vi "log.write_request.vi"(8 "error in":errorcluster, 9 "Arguments":map{string, string}(c390), 10 "Message":string, 11 "Time Stamp (now: system time)":timestamp format="%<%x %.3X>T") -> (0 "error out":errorcluster, 3 "request":string)   [LabVIEW 2020, in "Nominal Client.lvclass"]
uses:
  Nominal Client.lvclass
  4260bc31-df4d-47d5-a4e2-998131efb0a5.vi
  bb59544d-9623-4990-916d-6c8c801fc026.vi
  8accc981-0023-4d42-bd6a-63233f6e5657.vi
  <vilib>/LabVIEW Open Source Project/Epoch Date & Time/epoch.UNIX/Epoch.UNIX.lvclass
  C:/Program Files/National Instruments/LabVIEW 2020/vi.lib/LabVIEW Open Source Project/Epoch Date & Time/epoch/Epoch.lvclass
  <vilib>/LabVIEW Open Source Project/Epoch Date & Time/Get Epoch Time.vi
  <vilib>/JDP Science/JSONtext/Variant to JSON Text.vi
  <vilib>/JDP Science/JSONtext/support/Format JSON Object.vi
  <vilib>/JDP Science/JSONtext/LVClass Serializer/JSONtext LVClass Serializer.lvclass
  nominal types/properties/properties.lvclass
  Nominal Client.lvclass/Nominal Client.ctl
  <vilib>/JDP Science/JSONtext/JSONtext.lvlib
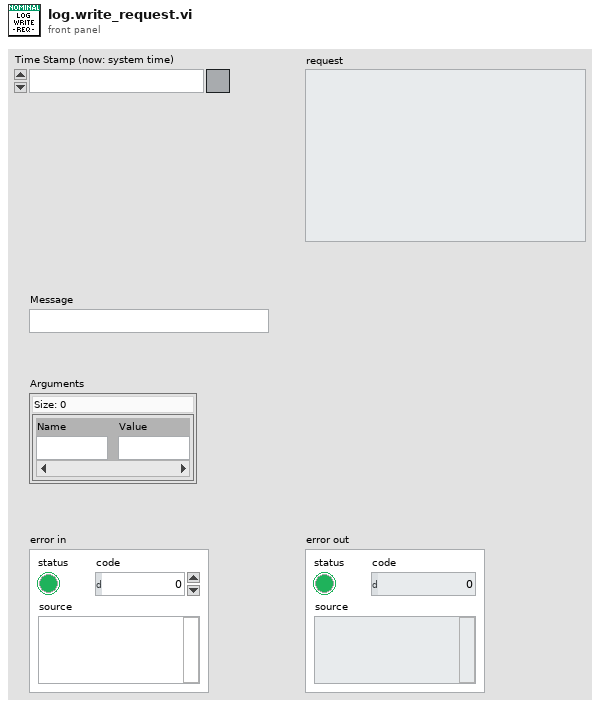
[diagram p1: front panel]
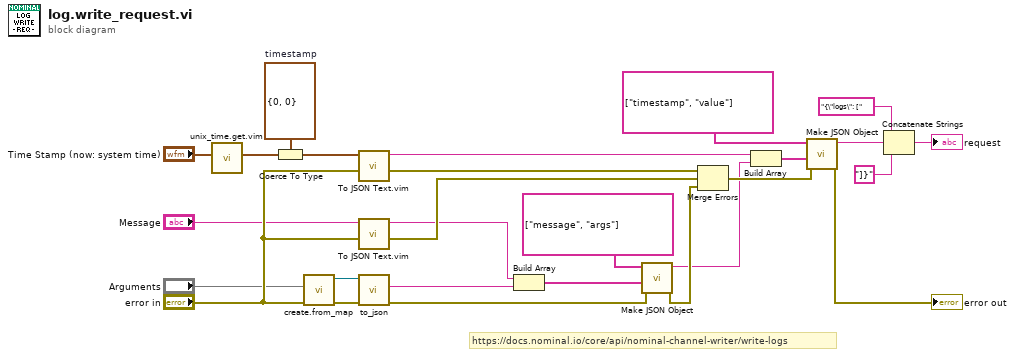
[diagram p0: block diagram]
diagram:
  w26 = cluster{"seconds":i32, "nanos":i32} {"seconds"=0, "nanos"=0}  # timestamp
  # "https://docs.nominal.io/core/api/nominal-channel-writer/write-logs"
  n1 = call "unix_time.get.vim"("Time Stamp (empty: now) [single or array]"="Time Stamp (now: system time)") -> ("UNIX Timestamp"=w27:cluster{"Seconds":i64, "Nanoseconds":i64})  [unwired: 10 in]
  n2 = Coerce To Type(0:w27, 1:w26) -> (2:w22:cluster{"seconds":i32, "nanos":i32})
  n3 = call "create.from_map.vi"("error in"="error in", "properties"="Arguments") -> ("error out"=w23:errorcluster, "properties out"=w24:refnum<class "properties.lvclass">)  [unwired: 8 in]
  n4 = call "To JSON Text.vim"("error in (no error)"="error in", "Anything"=w22) -> ("error out"=w10:errorcluster, "<JSON>"=w17:string)  [unwired: 8 in]
  n5 = call "To JSON Text.vim"("error in (no error)"="error in", "Anything"="Message") -> ("error out"=w9:errorcluster, "<JSON>"=w3:string)  [unwired: 8 in]
  n6 = call-dynamic "to_json.vi"("error in"=w23, "properties in"=w24) -> ("error out"=w11:errorcluster, "json"=w20:string)  [unwired: 6 in, 2 out]
  n7 = Build Array(w3, w20) -> (w19:string[])
  n8 = call <vilib>:"Make JSON Object.vi"("error in (no error)"=w11, "JSON Items"=w19, "Item Names"=string[] ["message", "args"]) -> ("error out"=w8:errorcluster, "<JSON>"=w6:string)  [unwired: 7 in]
  n9 = Merge Errors(w10, w9, w8) -> (w7:errorcluster)
  n10 = Build Array(w17, w6) -> (w16:string[])
  n11 = call <vilib>:"Make JSON Object.vi"("error in (no error)"=w7, "JSON Items"=w16, "Item Names"=string[] ["timestamp", "value"]) -> ("error out"=→"error out":errorcluster, "<JSON>"=w15:string)  [unwired: 7 in]
  n12 = Concatenate Strings("{\"logs\": [" ("string"), w15, "]}" ("string")) -> (→"request":string)
